vi "Auto - Commands.vi"(0 "Auton State In":i32, 9 "Auton Cluster In":T1) -> (1 "shoot":bool, 2 "suck":bool, 4 "Auton State Out":i32, 10 "Auton Cluster Out":T1, 12 "shooterSpinup":bool, 13 "spit":bool, 15 "disabledRunning":bool)   [LabVIEW 2020]
uses:
  TypeDefs/Auton Cluster Typedef.ctl
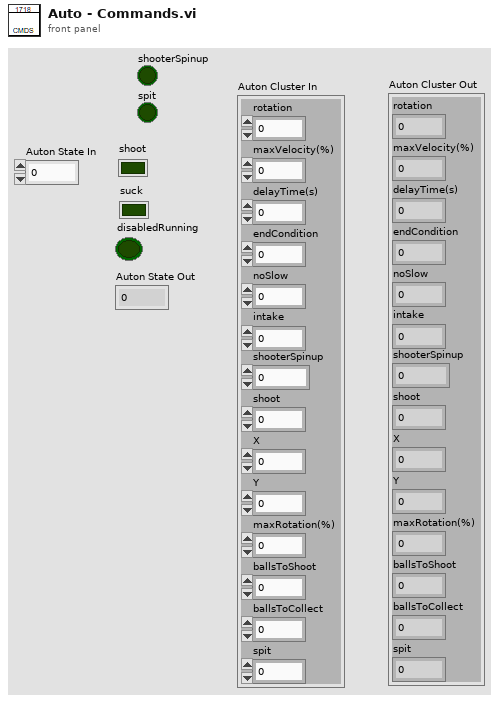
[diagram p1: front panel]
types:
  T1 = typedef "Auton Cluster Typedef.ctl" = cluster{"rotation":dbl, "maxVelocity(%)":dbl, "delayTime(s)":dbl, "endCondition":dbl, "noSlow":dbl, "intake":dbl, "shooterSpinup":dbl, "shoot":dbl, "X":dbl, "Y":dbl, "maxRotation(%)":dbl, "ballsToShoot":dbl, "ballsToCollect":dbl, "spit":dbl}
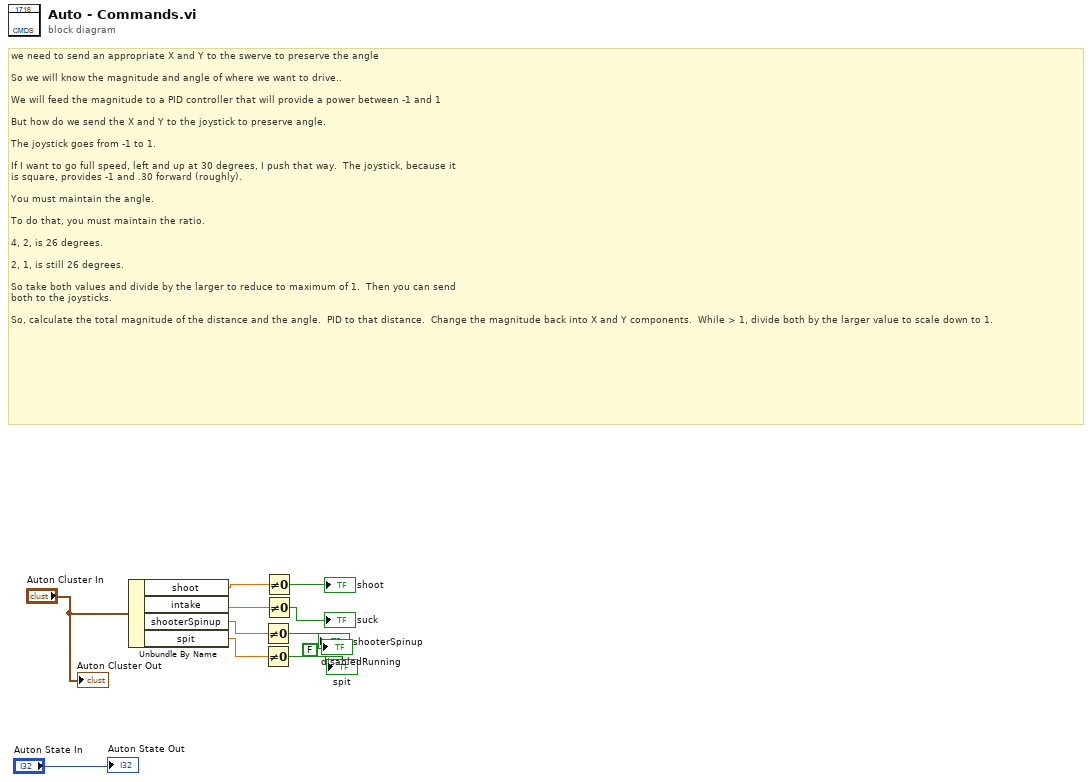
[diagram p0: block diagram]
diagram:
  # "we need to send an appropriate X and Y to the swerve to preserve the angle \n\nSo we will know the magnitude and angle of where we want to drive..\n\nWe will feed the magnitude to a PID controller that will provide a power between -1 and 1\n\nBut how do we send the X and Y to the joystick to preserve angle.\n\nThe joystick goes from -1 to 1.\n\nIf I want to go full speed, left and up at 30 degrees, I push that way.  The joystick, because it\nis square, provides -1 and .30 forward (roughly).\n\nYou must maintain the angle.\n\nTo do that, you must maintain the ratio.\n\n4, 2, is 26 degrees.\n\n2, 1, is still 26 degrees.\n\nSo take both values and divide by the larger to reduce to maximum of 1.  Then you can send\nboth to the joysticks.\n\nSo, calculate the total magnitude of the distance and the angle.  PID to that distance.  Change the magnitude back into X and Y components.  While > 1, divide both by the larger value to scale down to 1."
  n1 = Unbundle By Name("Auton Cluster In") -> ("shoot"=w9:dbl, "intake"=w8:dbl, "shooterSpinup"=w4:dbl, "spit"=w3:dbl)
  n2 = Not Equal To 0?(x=w4) -> (x != 0?=→"shooterSpinup":bool)
  n3 = Not Equal To 0?(x=w3) -> (x != 0?=→"spit":bool)
  n4 = Not Equal To 0?(x=w9) -> (x != 0?=→"shoot":bool)
  n5 = Not Equal To 0?(x=w8) -> (x != 0?=→"suck":bool)
  "Auton Cluster Out" <- "Auton Cluster In"
  "Auton State Out" <- "Auton State In"
  "disabledRunning" <- FALSE ("disabledRunning")
